vi "msg.vi"() -> (3 "data":string caption="데이터")   [LabVIEW 2014]
uses:
  <vilib>/FTP/NI_FTP.lvlib
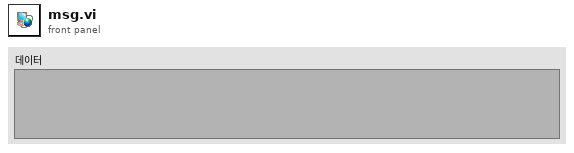
[diagram p1: front panel]
types:
  T1 = typedef "NI_FTP.lvlib/FTP Session.ctl" = refnum<k5>
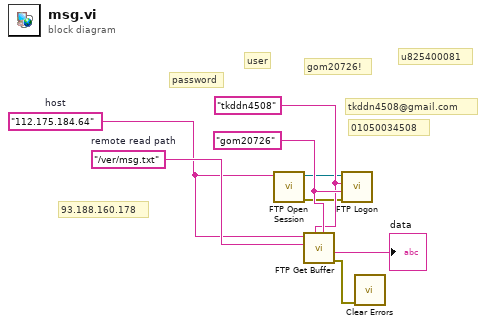
[diagram p0: block diagram]
diagram:
  w5 = "gom20726"
  w4 = "tkddn4508"
  w7 = "/ver/msg.txt"  # remote read path
  w6 = "112.175.184.64"  # host
  # "93.188.160.178"
  # "u825400081"
  # "gom20726!"
  # "01050034508"
  # "tkddn4508@gmail.com"
  # "user"
  # "password"
  n1 = call <vilib>:"FTP Open Session.vi"("address"=w6) -> ("error out"=w3:errorcluster, "ftp session"=w2:T1)  [unwired: 7 in, 2 out]
  n2 = call <vilib>:"FTP Get Buffer.vi"("password"=w5, "user"=w4, "remote path"=w7, "host"=w6) -> ("error out"=w1:errorcluster, "data"=→"data":string)  [unwired: 5 in, 1 out]
  n3 = call <vilib>:"FTP Logon.vi"("error in (no error)"=w3, "password"=w5, "user"=w4, "ftp session"=w2) -> ()  [unwired: 4 in, 4 out]
  n4 = call <vilib>:"Clear Errors.vi"("error in (no error)"=w1) -> ()  [unwired: 5 in, 2 out]
